vi "Get Display String.vi"(8 "error in":errorcluster, 11 "widget test\nresults in":refnum<class "Widget Test Results.lvclass">) -> (0 "error out":errorcluster, 2 "display string":string, 3 "widget test results out":refnum<class "Widget Test Results.lvclass">)   [LabVIEW 2020, in "Widget Test Results.lvclass"]
doc: "This VI is an example of a protected member VI of a LabVIEW class. Only VIs within the same class or a descendant class can call this VI. This is also an example of an override member VI."
uses:
  Widget Test Results.lvclass
  Widget Test Results.lvclass/Widget Test Results.ctl
  Test Results/Test Results Base Class.lvclass
panel:
  in  "widget ID \nformat string":string=" with widget id: %s"
  # "This VI is an example of a protected member VI of a LabVIEW class. \n\nThis is also an example of an override member VI."
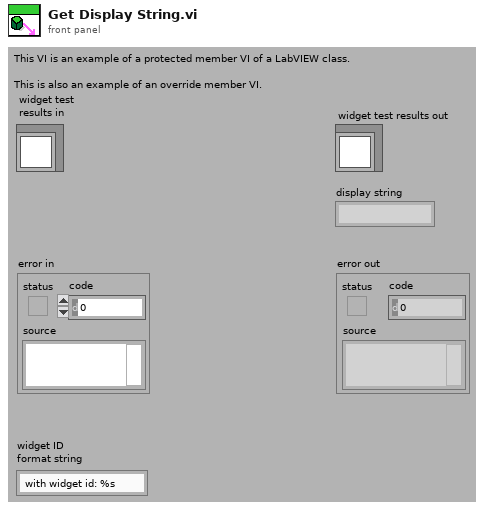
[diagram p1: front panel]
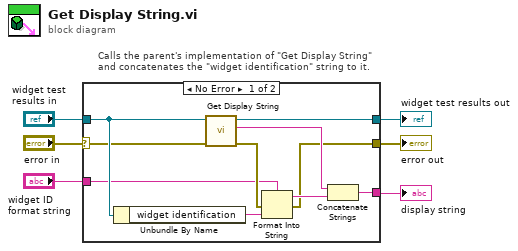
[diagram p0: block diagram]
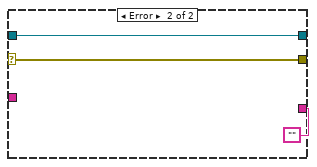
[diagram p2: hidden frame]
diagram:
  # "Calls the parent's implementation of \"Get Display String\" \nand concatenates the \"widget identification\" string to it."
  n1 = case shown="No Error" "error in" {
    selector: "error in" -> [w14 w18]
    tunnel: "widget test\nresults in" -> [w15 w19]
    tunnel: [w8 w18] -> w4
    tunnel: [w13 w19] -> w3
    tunnel: [w16 "" ("Empty String Constant")] -> w2
    tunnel: "widget ID \nformat string" -> [w7 _]
    frame No Error {
      n2 = Unbundle By Name(w15) -> ("widget identification"=w11:string)
      n3 = call-parent "Get Display String.vi"("error in"=w14, "test\nresults in"=w15) -> ("error out"=w9:errorcluster, "display string"=w12:string, "test results out"=w13:refnum<class "Widget Test Results.lvclass">)  [unwired: 7 in]
      n4 = Format Into String(format string=w7, error in=w9, w11) -> (resulting string=w10:string, error out=w8:errorcluster)  [unwired: 1 in]
      n5 = Concatenate Strings(w12, w10) -> (w16:string)
    }
    frame Error {
    }
  }
  "error out" <- w4
  "display string" <- w2
  "widget test results out" <- w3
